vi "Init session.vi"(8 "error in (no error)":errorcluster {"code" format="%.0x"}, 9 "Simulate":bool=TRUE, 10 "option string":string, 11 "resource string":refnum<visa-resource-name>="USB0::0x0957::0x1798::MY52161667::INSTR") -> (0 "error out":errorcluster {"code" format="%.0x"}, 2 "log string out":string, 3 "instrument handle out":refnum<k15>)   [LabVIEW 2021]
uses:
  <instrlib>/Keysight InfiniiVision/Keysight InfiniiVision.lvlib
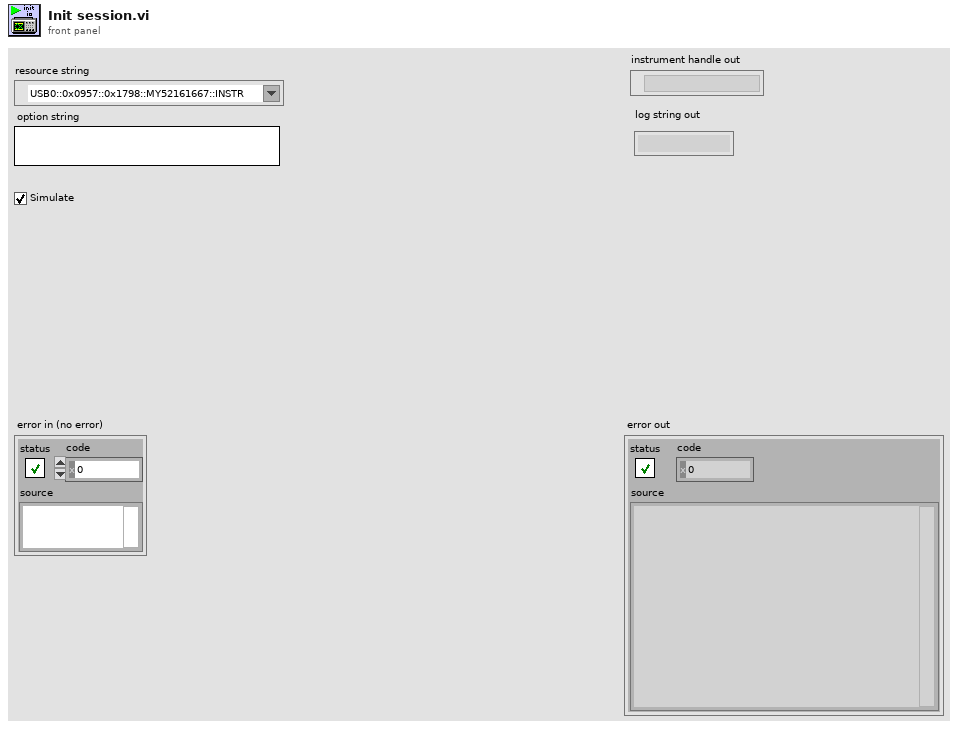
[diagram p1: front panel]
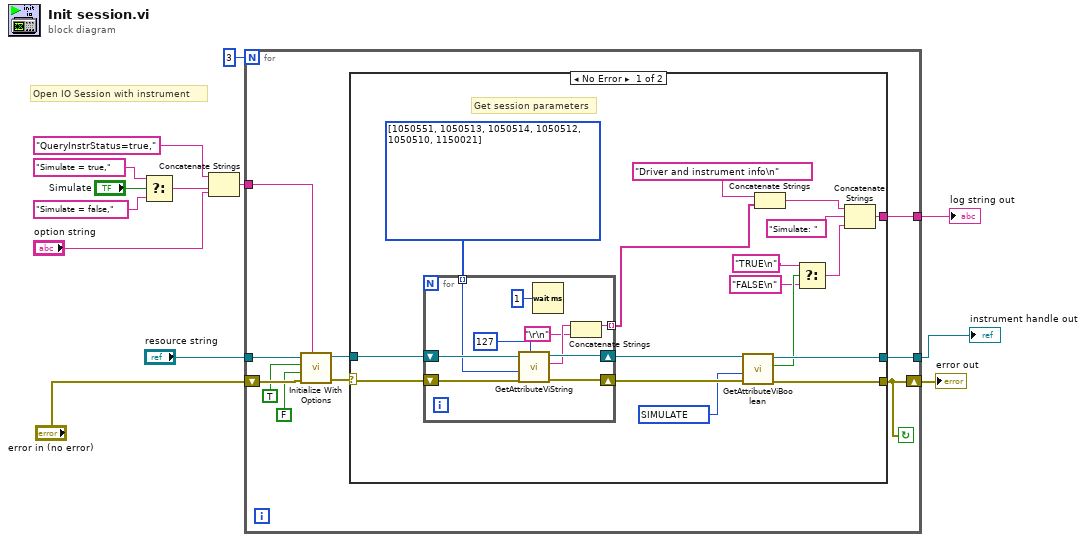
[diagram p0: block diagram]
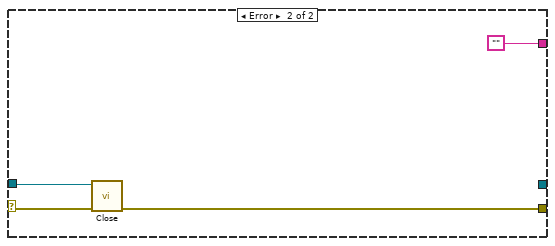
[diagram p2: hidden frame]
diagram:
  # "Open IO Session with instrument"
  n1 = Select(t="Simulate = true,", s="Simulate", f="Simulate = false,") -> (s? t:f=w3:string)
  n2 = Concatenate Strings("QueryInstrStatus=true," ("string"), w3, "option string") -> (w1:string)
  n3 = for {
    N: 3 -> [_]
    tunnel: [w19] -> w7
    shift-right: [w15] -> w10
    shift-left: "error in (no error)" -> [w20]
    tunnel: "resource string" -> [w16]
    tunnel: [w21] -> w9
    tunnel: w1 -> [w14]
    stop <- w15 continue-if-true
    n4 = call <instrlib>:"Initialize With Options.vi"("option string"=w14, "error in (no error)"=w20, "reset device (Off)"=FALSE ("id query (Off)"), "id query (Off)"=TRUE, "resource string"=w16) -> ("error out"=w22:errorcluster, "instrument handle out"=w23:refnum<k15>)  [unwired: 5 in]
    n5 = case shown="No Error" w22 {
      selector: w22 -> [w38 w52]
      tunnel: w23 -> [w39 w53]
      tunnel: [w33 w51] -> w15
      tunnel: [w34 _] -> w21
      tunnel: [w24 ""] -> w19
      frame No Error {
        w36 = u32 1050005 items=["CHANNEL_ENABLED"=1250005, "CHANNEL_INVERT"=1150026, "DIGITALCHANNEL_ENABLED"=1150039, "DVM_AUTO_RANGE_ENABLED"=1150439, "DVM_ENABLED"=1150441, "INITIATE_CONTINUOUS"=1250107, "SIMULATE"=1050005, "STATISTICS_DISPLAY_ENABLED"=1150430, "STATISTICS_RELATIVE_STD_DEV_ENABLED"=1150357, "SYSTEM_PRECISION_ENABLED"=1150588, "SYSTEM_PROTECTION_ENABLED"=1150130, "SYSTEM_TOUCH_SCREEN_ENABLED"=1150514, "SYSTEM_TRACE_ENABLED"=1150024, "TIMEBASE_VERNIER_ENABLED"=1150112, "TRIGGER_HF_REJECT_FILTER_ENABLED"=1150137, "TRIGGER_NOISE_REJECT_FILTER_ENABLED"=1150136, "UNSIGNED_MODE_ENABLE"=1150092] ("AttributeID")
        w40 = u32[] [1050551, 1050513, 1050514, 1050512, 1050510, 1150021] items=["CHANNEL_LABEL"=1150027, "CHANNEL_PROBEID"=1150029, "DIGITALCHANNEL_LABEL"=1150040, "DIGITALCHANNEL_THRESHOLD"=1150043, "DRIVER_SETUP"=1050007, "DVM_SOURCE"=1150444, "INSTRUMENT_FIRMWARE_REVISION"=1050510, "INSTRUMENT_MANUFACTURER"=1050511, "INSTRUMENT_MODEL"=1050512, "IO_RESOURCE_DESCRIPTOR"=1050304, "LOGICAL_NAME"=1050305, "SPECIFIC_DRIVER_DESCRIPTION"=1050514, "SPECIFIC_DRIVER_REVISION"=1050551, "SPECIFIC_DRIVER_VENDOR"=1050513, "STATISTICS_COUNT"=1150356, "SUPPORTED_INSTRUMENT_MODELS"=1050327, "SYSTEM_SERIAL_NUMBER"=1150021, "SYSTEM_SYSTEM_DATE"=1150020, "SYSTEM_TIME"=1150022, "TRIGGER_DELAY_ARMING_SOURCE"=1150264, "TRIGGER_OR_EDGE_PATTERN"=1150262, "TRIGGER_PATTERN_ANALOG_PATTERN"=1150193, "TRIGGER_PATTERN_DIGITAL_PATTERN"=1150194, "TRIGGER_SETUP_AND_HOLD_CLOCK_SOURCE"=1150253, "TRIGGER_SETUP_AND_HOLD_DATA_SOURCE"=1150254, "TRIGGER_SOURCE"=1250013, "TRIGGER_ZONE_SOURCE"=1150468, "VIEW"=1150142, "WAVEFORM_SOURCE"=1150091]
        # "Get session parameters"
        n6 = for {
          shift-right: [w48] -> w35
          shift-left: w39 -> [w49]
          shift-right: [w46] -> w37
          shift-left: w38 -> [w47]
          tunnel: w40 -> [w44] mode=indexing
          tunnel: [w42] -> w30 mode=indexing
          n7 = call <instrlib>:"GetAttributeViString.vi"("AttributeValueBufferSize"=127, "error in (no error)"=w47, "AttributeID"=w44, "instrument handle"=w49) -> ("error out"=w46:errorcluster, "AttributeValue"=w43:string, "instrument handle out"=w48:refnum<k15>)  [unwired: 5 in]
          n8 = Wait (ms)(milliseconds to wait=u32 1) -> ()  [unwired: 1 out]
          n9 = Concatenate Strings(w43, "\r\n") -> (w42:string)
        }
        n10 = call <instrlib>:"GetAttributeViBoolean.vi"("error in (no error)"=w37, "AttributeID"=w36, "instrument handle"=w35) -> ("error out"=w33:errorcluster, "AttributeValue"=w31:bool, "instrument handle out"=w34:refnum<k15>)  [unwired: 6 in]
        n11 = Concatenate Strings("Driver and instrument info\n" ("string"), w30) -> (w25:string)
        n12 = Select(t="TRUE\n", s=w31, f="FALSE\n") -> (s? t:f=w27:string)
        n13 = Concatenate Strings(w25, "Simulate: " ("string"), w27) -> (w24:string)
      }
      frame Error {
        n14 = call <instrlib>:"Close.vi"("error in (no error)"=w52, "instrument handle"=w53) -> ("error out"=w51:errorcluster)  [unwired: 9 in]
      }
    }
  }
  "instrument handle out" <- w9
  "error out" <- w10
  "log string out" <- w7
